vi "Write Stabilization Data.vi"(8 "error in (no error)":errorcluster, 10 "Metadata Cluster":T1, 11 "Stabilization Data":T2={"Stabilization waveform"={"t0"=timestamp(0 s since 1904-01-01), "dt"=50.0, "Y"=[10.0, 9.0, 8.75, 8.5, 8.25, 8.125, 8.06, 8.03, 8.015, 8.0, 8.0, 8.0]}, "Variation"=0.0, "Stabilized"=FALSE, "Threshold"=0.0, "time to stabilize"=0.0, "3 points"=[], "Sphere Indicator"=enum."Naked Sphere"}) -> (0 "error out":errorcluster)   [LabVIEW 2013]
uses:
  Timing and Stabilization/Stabilization.ctl
  avantesSpectrometer/Acquisition/Sphere Indicator.ctl
  Metadata Cluster.ctl
  avantesSpectrometer/AvaSpec.lvlib
  Timing and Stabilization.lvlib
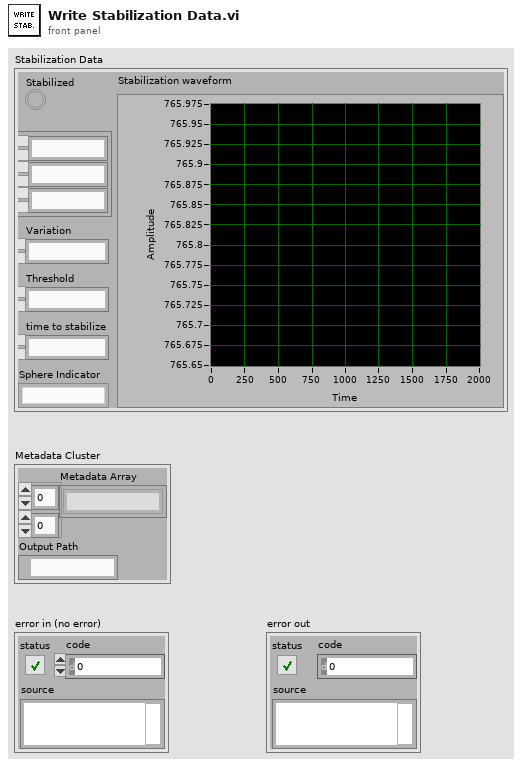
[diagram p1: front panel]
types:
  T1 = typedef "Metadata Cluster.ctl" = cluster{"Metadata Array":string[][], "Output Path":path}
  T2 = typedef "Timing and Stabilization.lvlib/Stabilization.ctl" = cluster{"Stabilization waveform":waveform(dbl), "Variation":dbl, "Stabilized":bool, "Threshold":dbl, "time to stabilize":dbl, "3 points":dbl[], "Sphere Indicator":T3}
  T3 = typedef "AvaSpec.lvlib/Sphere Indicator.ctl" = enum16{"Naked Sphere", "Insulated Sphere"}
  T4 = enum16{"open", "open or create", "create or replace", "create", "open (read-only)"}
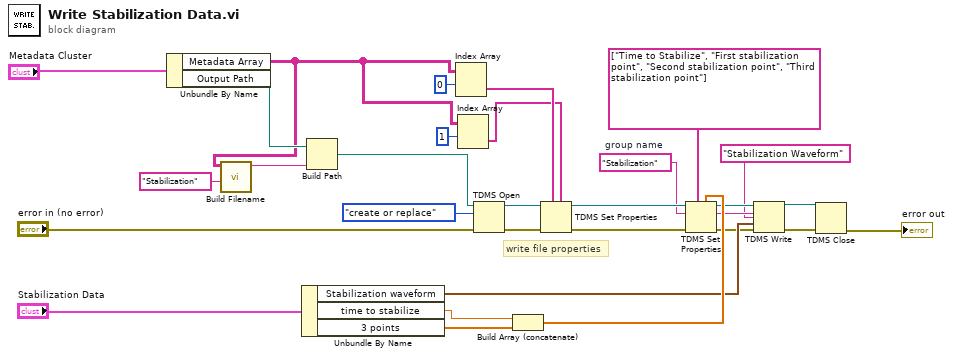
[diagram p0: block diagram]
diagram:
  w6 = "Stabilization"  # group name
  # "write file properties"
  n1 = Unbundle By Name("Metadata Cluster") -> ("Metadata Array"=w2:string[][], "Output Path"=w4:path)
  n2 = call "Build Filename.vi"("Measurment Type"="Stabilization", "Metadata In"=w2) -> ("String"=w22:string)  [unwired: 9 in]
  n3 = Unbundle By Name("Stabilization Data") -> ("Stabilization waveform"=w26:waveform(dbl), "time to stabilize"=w29:dbl, "3 points"=w28:dbl[])
  n4 = Build Path(base path=w4, name or relative path=w22) -> (appended path=w10:path)
  n5 = Index Array(array=w2, index (row)=0) -> (element=w12:string[])  [unwired: 1 in]
  n6 = Index Array(array=w2, index (row)=1) -> (element=w11:string[])  [unwired: 1 in]
  n7 = TDMS Open(8:"error in (no error)", 10:T4."create or replace" ("operation (0:open)"), 11:w10) -> (0:w21:errorcluster, 3:w19:refnum<k34>)  [unwired: 4 in]
  n8 = Build Array (concatenate)(w29, w28) -> (w27:dbl[])
  n9 = TDMS Set Properties(5:w11, 7:w12, 8:w21, 11:w19) -> (0:w15:errorcluster, 3:w16:refnum<k34>)  [unwired: 2 in, 2 out]
  n10 = TDMS Set Properties(5:w27, 7:string[] ["Time to Stabilize", "First stabilization point", "Second stabilization point", "Third stabilization point"] ("property names"), 8:w15, 10:w6, 11:w16) -> (0:w8:errorcluster, 2:w9:string, 3:w7:refnum<k34>)  [unwired: 1 in, 1 out]
  n11 = TDMS Write(0:w7, 5:w9, 7:"Stabilization Waveform" ("channel name(s) in (Untitled)"), 9:w26, 11:w8) -> (4:w18:refnum<k34>, 15:w17:errorcluster)  [unwired: 1 in, 2 out]
  n12 = TDMS Close(8:w17, 11:w18) -> (0:→"error out":errorcluster)  [unwired: 1 out]
